vi "rigol-dp832.vi"() -> ()   [LabVIEW 2024]
uses:
  <vilib>/Instr/_visa.llb/VISA Open Access Mode.ctl
panel:
  out "CH1_on 3":bool
  out "CH1_on 2":bool
  out "CH1_on":bool
  out "CH1 Voltage 3":string
  out "CH1 Current 3":string
  out "CH1 Voltage 2":string
  out "CH1 Current 2":string
  out "CH1 Current":string
  in  "stop":bool
  out "error out":errorcluster
  out "CH1 Voltage":string
  in  "error in (no error)":errorcluster
  in  "VISA resource name":refnum<visa-resource-name>="TCPIP0::172.16.15.121::inst0::INSTR"
  # "CH1"
  # "CH2"
  # "CH3"
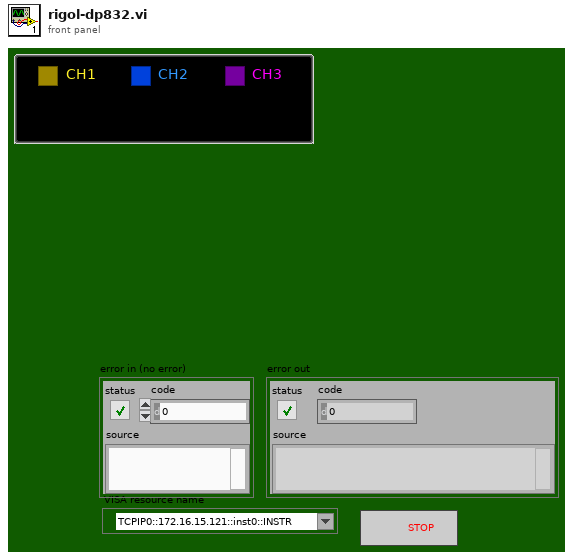
[diagram p1: front panel]
types:
  T1 = typedef "VISA Open Access Mode.ctl" = u32
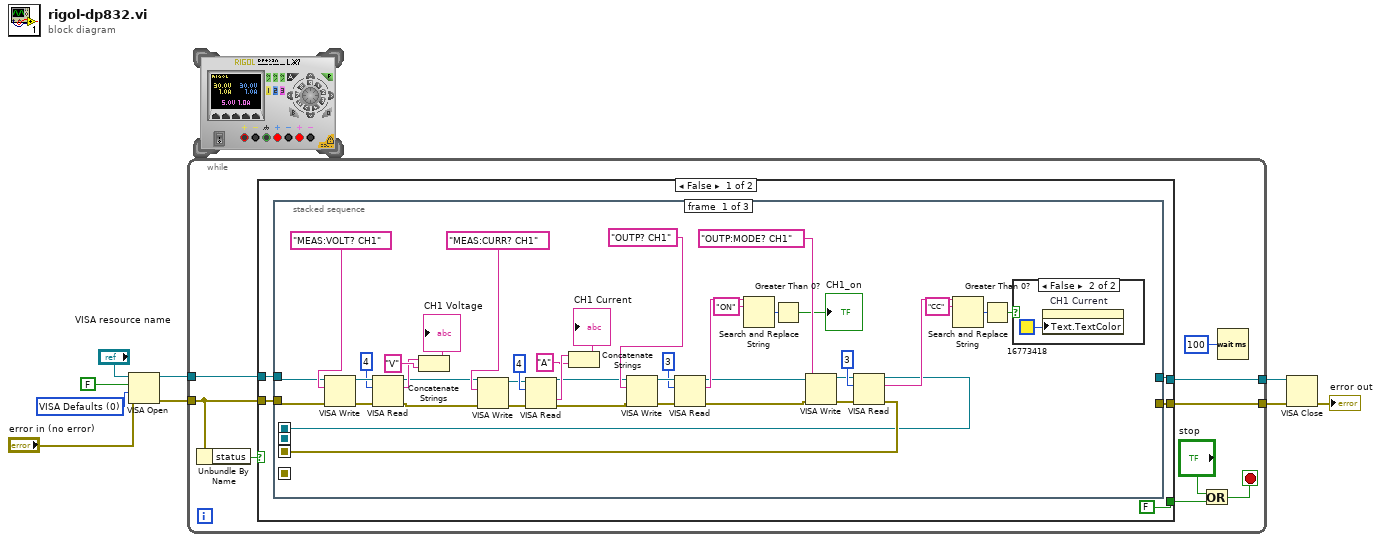
[diagram p0: block diagram]
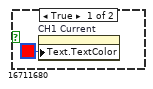
[diagram p2: hidden frame]
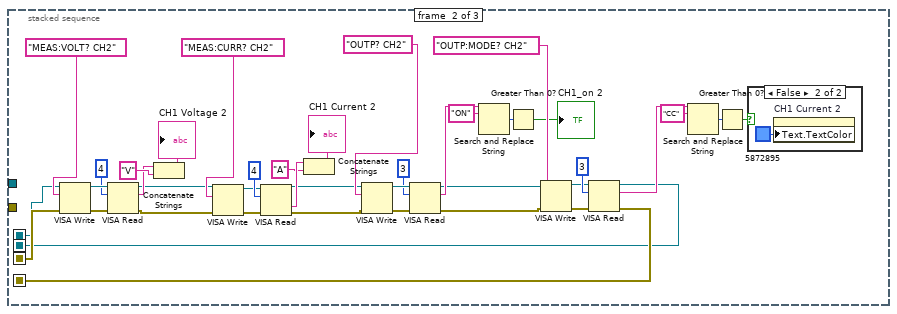
[diagram p3: hidden frame]
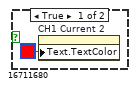
[diagram p4: hidden frame]
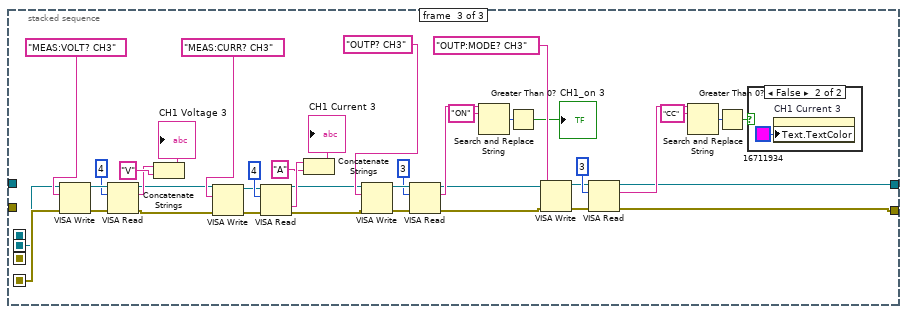
[diagram p5: hidden frame]
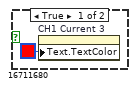
[diagram p6: hidden frame]
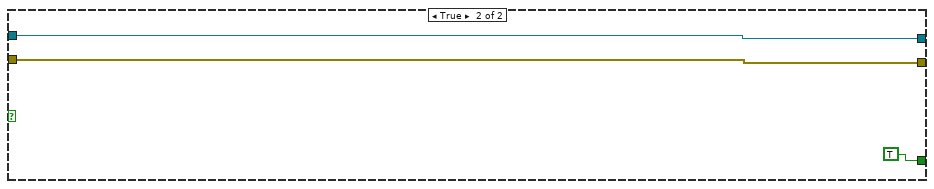
[diagram p7: hidden frame]
diagram:
  w7 = T1 0 items=["VISA Defaults"=0, "Exclusive Lock"=1, "Load Configured Settings"=4] ("Access Mode")
  n1 = VISA Open(duplicate session (F)=FALSE, access mode=w7, error in (no error)="error in (no error)", VISA resource name="VISA resource name") -> (VISA resource name=w4:refnum<visa-resource-name>, error out=w5:errorcluster)  [unwired: 1 in]
  n2 = while {
    tunnel: w5 -> [w14]
    tunnel: w4 -> [w17]
    tunnel: [w15] -> w2
    tunnel: [w16] -> w1
    stop <- w11 stop-if-true
    n3 = Unbundle By Name(w14) -> ("status"=w13:bool)
    n4 = case shown="False" w13 {
      tunnel: w17 -> [w23 w152]
      tunnel: [w21 w152] -> w16
      tunnel: [w20 w151] -> w15
      tunnel: w14 -> [w22 w151]
      tunnel: [FALSE TRUE] -> w10
      frame False {
        n5 = stacked-sequence {
          seq-local: [w26 _ _] -> [_ w70 _]
          seq-local: [_ w69 _] -> [_ _ w112]
          seq-local: [w25 _ _] -> [_ w67 _]
          seq-local: [_ w68 _] -> [_ _ w110]
          tunnel: w23 -> [w59 _ _]
          tunnel: w22 -> [w58 _ _]
          tunnel: [_ _ w109] -> w21
          tunnel: [_ _ w111] -> w20
          frame #0 {
            n6 = VISA Write(VISA resource name=w59, write buffer="MEAS:VOLT? CH1" ("write buffer voltage"), error in (no error)=w58) -> (VISA resource name out=w61:refnum<visa-resource-name>, error out=w62:errorcluster)  [unwired: 1 out]
            n7 = VISA Read(VISA resource name=w61, byte count=u32 4, error in (no error)=w62) -> (VISA resource name out=w50:refnum<visa-resource-name>, read buffer=w51:string, error out=w48:errorcluster)  [unwired: 1 out]
            n8 = Concatenate Strings(w51, "V" ("string")) -> (→"CH1 Voltage":string)
            n9 = VISA Write(VISA resource name=w50, write buffer="MEAS:CURR? CH1" ("write buffer voltage"), error in (no error)=w48) -> (VISA resource name out=w56:refnum<visa-resource-name>, error out=w49:errorcluster)  [unwired: 1 out]
            n10 = VISA Read(VISA resource name=w56, byte count=u32 4, error in (no error)=w49) -> (VISA resource name out=w43:refnum<visa-resource-name>, read buffer=w54:string, error out=w42:errorcluster)  [unwired: 1 out]
            n11 = Concatenate Strings(w54, "A" ("string")) -> (→"CH1 Current":string)
            n12 = VISA Write(VISA resource name=w43, write buffer="OUTP? CH1" ("write buffer voltage"), error in (no error)=w42) -> (VISA resource name out=w45:refnum<visa-resource-name>, error out=w47:errorcluster)  [unwired: 1 out]
            n13 = VISA Read(VISA resource name=w45, byte count=u32 3, error in (no error)=w47) -> (VISA resource name out=w33:refnum<visa-resource-name>, read buffer=w41:string, error out=w34:errorcluster)  [unwired: 1 out]
            n14 = Search and Replace String(input string=w41, search string="ON") -> (number of replacements=w39:i32)  [unwired: 6 in, 3 out]
            n15 = Greater Than 0?(x=w39) -> (x > 0?=→"CH1_on":bool)
            n16 = VISA Write(VISA resource name=w33, write buffer="OUTP:MODE? CH1" ("write buffer voltage"), error in (no error)=w34) -> (VISA resource name out=w37:refnum<visa-resource-name>, error out=w35:errorcluster)  [unwired: 1 out]
            n17 = VISA Read(VISA resource name=w37, byte count=u32 3, error in (no error)=w35) -> (VISA resource name out=w25:refnum<visa-resource-name>, read buffer=w29:string, error out=w26:errorcluster)  [unwired: 1 out]
            n18 = Search and Replace String(input string=w29, search string="CC") -> (number of replacements=w31:i32)  [unwired: 6 in, 3 out]
            n19 = Greater Than 0?(x=w31) -> (x > 0?=w32:bool)
            n20 = case shown="False" w32 {
              frame True {
                n21 = property on="CH1 Current" class="Str"("Text.TextColor"=u32 16711680 ("Text.Colors:FG Color")) -> ()  [unwired: 2 in, 2 out]
              }
              frame False {
                n22 = property on="CH1 Current" class="Str"("Text.TextColor"=u32 16773418 ("Text.Colors:FG Color")) -> ()  [unwired: 2 in, 2 out]
              }
            }
          }
          frame #1 {
            n23 = VISA Write(VISA resource name=w67, write buffer="MEAS:VOLT? CH2" ("write buffer voltage"), error in (no error)=w70) -> (VISA resource name out=w103:refnum<visa-resource-name>, error out=w104:errorcluster)  [unwired: 1 out]
            n24 = VISA Read(VISA resource name=w103, byte count=u32 4, error in (no error)=w104) -> (VISA resource name out=w94:refnum<visa-resource-name>, read buffer=w95:string, error out=w92:errorcluster)  [unwired: 1 out]
            n25 = Concatenate Strings(w95, "V" ("string")) -> (→"CH1 Voltage 2":string)
            n26 = VISA Write(VISA resource name=w94, write buffer="MEAS:CURR? CH2" ("write buffer voltage"), error in (no error)=w92) -> (VISA resource name out=w100:refnum<visa-resource-name>, error out=w93:errorcluster)  [unwired: 1 out]
            n27 = VISA Read(VISA resource name=w100, byte count=u32 4, error in (no error)=w93) -> (VISA resource name out=w87:refnum<visa-resource-name>, read buffer=w98:string, error out=w86:errorcluster)  [unwired: 1 out]
            n28 = Concatenate Strings(w98, "A" ("string")) -> (→"CH1 Current 2":string)
            n29 = VISA Write(VISA resource name=w87, write buffer="OUTP? CH2" ("write buffer voltage"), error in (no error)=w86) -> (VISA resource name out=w89:refnum<visa-resource-name>, error out=w91:errorcluster)  [unwired: 1 out]
            n30 = VISA Read(VISA resource name=w89, byte count=u32 3, error in (no error)=w91) -> (VISA resource name out=w77:refnum<visa-resource-name>, read buffer=w85:string, error out=w78:errorcluster)  [unwired: 1 out]
            n31 = Search and Replace String(input string=w85, search string="ON") -> (number of replacements=w83:i32)  [unwired: 6 in, 3 out]
            n32 = Greater Than 0?(x=w83) -> (x > 0?=→"CH1_on 2":bool)
            n33 = VISA Write(VISA resource name=w77, write buffer="OUTP:MODE? CH2" ("write buffer voltage"), error in (no error)=w78) -> (VISA resource name out=w81:refnum<visa-resource-name>, error out=w79:errorcluster)  [unwired: 1 out]
            n34 = VISA Read(VISA resource name=w81, byte count=u32 3, error in (no error)=w79) -> (VISA resource name out=w68:refnum<visa-resource-name>, read buffer=w73:string, error out=w69:errorcluster)  [unwired: 1 out]
            n35 = Search and Replace String(input string=w73, search string="CC") -> (number of replacements=w75:i32)  [unwired: 6 in, 3 out]
            n36 = Greater Than 0?(x=w75) -> (x > 0?=w76:bool)
            n37 = case shown="False" w76 {
              frame True {
                n38 = property on="CH1 Current 2" class="Str"("Text.TextColor"=u32 16711680 ("Text.Colors:FG Color")) -> ()  [unwired: 2 in, 2 out]
              }
              frame False {
                n39 = property on="CH1 Current 2" class="Str"("Text.TextColor"=u32 5872895 ("Text.Colors:FG Color")) -> ()  [unwired: 2 in, 2 out]
              }
            }
          }
          frame #2 {
            n40 = VISA Write(VISA resource name=w110, write buffer="MEAS:VOLT? CH3" ("write buffer voltage"), error in (no error)=w112) -> (VISA resource name out=w145:refnum<visa-resource-name>, error out=w146:errorcluster)  [unwired: 1 out]
            n41 = VISA Read(VISA resource name=w145, byte count=u32 4, error in (no error)=w146) -> (VISA resource name out=w136:refnum<visa-resource-name>, read buffer=w137:string, error out=w134:errorcluster)  [unwired: 1 out]
            n42 = Concatenate Strings(w137, "V" ("string")) -> (→"CH1 Voltage 3":string)
            n43 = VISA Write(VISA resource name=w136, write buffer="MEAS:CURR? CH3" ("write buffer voltage"), error in (no error)=w134) -> (VISA resource name out=w142:refnum<visa-resource-name>, error out=w135:errorcluster)  [unwired: 1 out]
            n44 = VISA Read(VISA resource name=w142, byte count=u32 4, error in (no error)=w135) -> (VISA resource name out=w129:refnum<visa-resource-name>, read buffer=w140:string, error out=w128:errorcluster)  [unwired: 1 out]
            n45 = Concatenate Strings(w140, "A" ("string")) -> (→"CH1 Current 3":string)
            n46 = VISA Write(VISA resource name=w129, write buffer="OUTP? CH3" ("write buffer voltage"), error in (no error)=w128) -> (VISA resource name out=w131:refnum<visa-resource-name>, error out=w133:errorcluster)  [unwired: 1 out]
            n47 = VISA Read(VISA resource name=w131, byte count=u32 3, error in (no error)=w133) -> (VISA resource name out=w119:refnum<visa-resource-name>, read buffer=w127:string, error out=w120:errorcluster)  [unwired: 1 out]
            n48 = Search and Replace String(input string=w127, search string="ON") -> (number of replacements=w125:i32)  [unwired: 6 in, 3 out]
            n49 = Greater Than 0?(x=w125) -> (x > 0?=→"CH1_on 3":bool)
            n50 = VISA Write(VISA resource name=w119, write buffer="OUTP:MODE? CH3" ("write buffer voltage"), error in (no error)=w120) -> (VISA resource name out=w123:refnum<visa-resource-name>, error out=w121:errorcluster)  [unwired: 1 out]
            n51 = VISA Read(VISA resource name=w123, byte count=u32 3, error in (no error)=w121) -> (VISA resource name out=w109:refnum<visa-resource-name>, read buffer=w115:string, error out=w111:errorcluster)  [unwired: 1 out]
            n52 = Search and Replace String(input string=w115, search string="CC") -> (number of replacements=w117:i32)  [unwired: 6 in, 3 out]
            n53 = Greater Than 0?(x=w117) -> (x > 0?=w118:bool)
            n54 = case shown="False" w118 {
              frame True {
                n55 = property on="CH1 Current 3" class="Str"("Text.TextColor"=u32 16711680 ("Text.Colors:FG Color")) -> ()  [unwired: 2 in, 2 out]
              }
              frame False {
                n56 = property on="CH1 Current 3" class="Str"("Text.TextColor"=u32 16711934 ("Text.Colors:FG Color")) -> ()  [unwired: 2 in, 2 out]
              }
            }
          }
        }
      }
      frame True {
      }
    }
    n57 = Or(x="stop", y=w10) -> (x .or. y?=w11:bool)
    n58 = Wait (ms)(milliseconds to wait=u32 100) -> ()  [unwired: 1 out]
  }
  n59 = VISA Close(VISA resource name=w1, error in (no error)=w2) -> (error out=→"error out":errorcluster)
